vi "log.write.request.vi"(6 "Channel":string, 8 "error in":errorcluster, 9 "Arguments":map{string, string}(c390), 10 "Message":string, 11 "Time Stamp (now: system time)":timestamp format="%<%x %.3X>T") -> (0 "error out":errorcluster, 3 "request":string)   [LabVIEW 2020, in "Nominal Client.lvclass"]
uses:
  Nominal Client.lvclass
  8accc981-0023-4d42-bd6a-63233f6e5657.vi
  4260bc31-df4d-47d5-a4e2-998131efb0a5.vi
  bb59544d-9623-4990-916d-6c8c801fc026.vi
  9ae5cbee-81e9-4394-a3ea-0608fb529230.vi
  <vilib>/LabVIEW Open Source Project/Epoch Date & Time/epoch.UNIX/Epoch.UNIX.lvclass
  C:/Program Files (x86)/National Instruments/LabVIEW 2020/vi.lib/LabVIEW Open Source Project/Epoch Date & Time/epoch/Epoch.lvclass
  <vilib>/LabVIEW Open Source Project/Epoch Date & Time/Get Epoch Time.vi
  <vilib>/JDP Science/JSONtext/Variant to JSON Text.vi
  <vilib>/JDP Science/JSONtext/support/Format JSON Object.vi
  <vilib>/JDP Science/JSONtext/support/Format JSON Array Text.vi
  <vilib>/JDP Science/JSONtext/LVClass Serializer/JSONtext LVClass Serializer.lvclass
  nominal types/properties/properties.lvclass
  <vilib>/JDP Science/JSONtext/JSONtext.lvlib
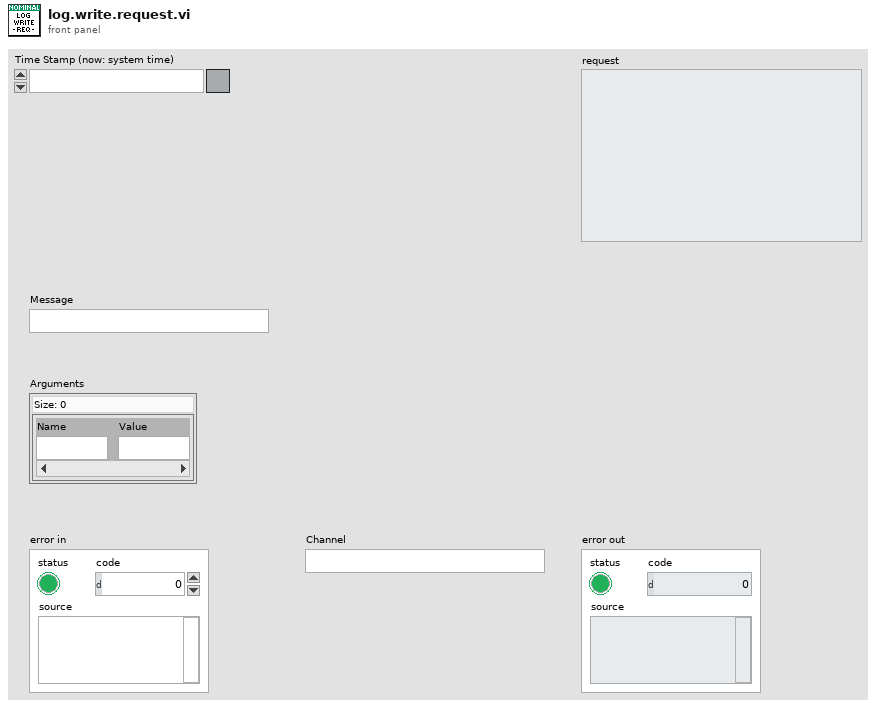
[diagram p1: front panel]
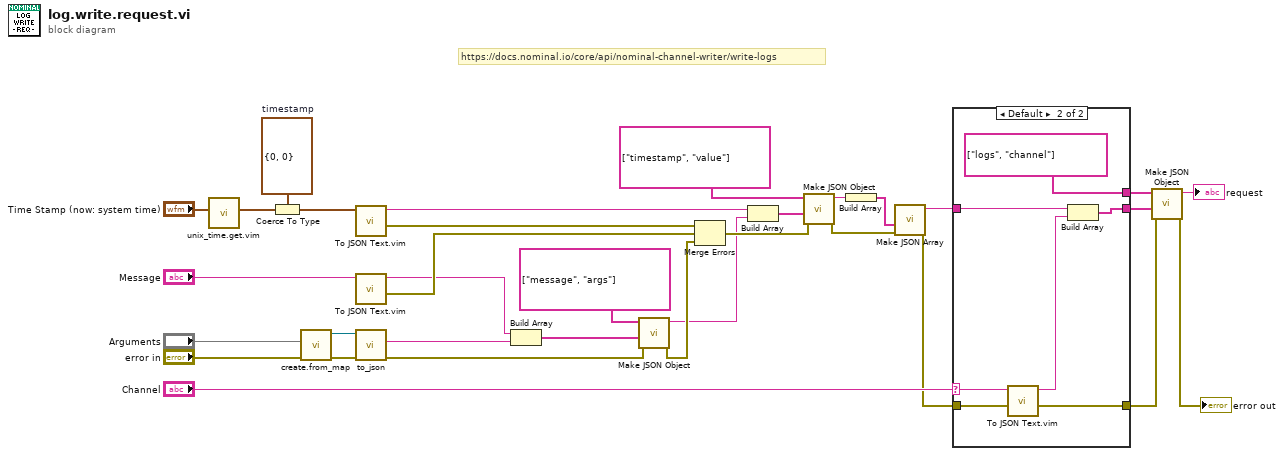
[diagram p0: block diagram]
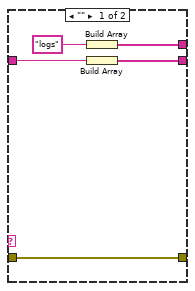
[diagram p2: hidden frame]
diagram:
  w32 = cluster{"seconds":i32, "nanos":i32} {"seconds"=0, "nanos"=0}  # timestamp
  # "https://docs.nominal.io/core/api/nominal-channel-writer/write-logs"
  n1 = call "unix_time.get.vim"("Time Stamp (empty: now) [single or array]"="Time Stamp (now: system time)") -> ("UNIX Timestamp"=w33:cluster{"Seconds":i64, "Nanoseconds":i64})  [unwired: 10 in]
  n2 = Coerce To Type(0:w33, 1:w32) -> (2:w28:cluster{"seconds":i32, "nanos":i32})
  n3 = call "create.from_map.vi"("error in"="error in", "properties"="Arguments") -> ("error out"=w29:errorcluster, "properties out"=w30:refnum<class "properties.lvclass">)  [unwired: 8 in]
  n4 = call "To JSON Text.vim"("Anything"=w28) -> ("error out"=w19:errorcluster, "<JSON>"=w23:string)  [unwired: 9 in]
  n5 = call "To JSON Text.vim"("Anything"="Message") -> ("error out"=w18:errorcluster, "<JSON>"=w14:string)  [unwired: 9 in]
  n6 = call-dynamic "to_json.vi"("error in"=w29, "properties in"=w30) -> ("error out"=w20:errorcluster, "json"=w26:string)  [unwired: 6 in, 2 out]
  n7 = Build Array(w14, w26) -> (w25:string[])
  n8 = call <vilib>:"Make JSON Object.vi"("error in (no error)"=w20, "JSON Items"=w25, "Item Names"=string[] ["message", "args"]) -> ("error out"=w17:errorcluster, "<JSON>"=w15:string)  [unwired: 7 in]
  n9 = Merge Errors(w19, w18, w17) -> (w16:errorcluster)
  n10 = Build Array(w23, w15) -> (w22:string[])
  n11 = call <vilib>:"Make JSON Object.vi"("error in (no error)"=w16, "JSON Items"=w22, "Item Names"=string[] ["timestamp", "value"]) -> ("error out"=w6:errorcluster, "<JSON>"=w9:string)  [unwired: 7 in]
  n12 = Build Array(w9) -> (w10:string[])
  n13 = call <vilib>:"Make JSON Array.vi"("error in (no error)"=w6, "JSON Elements"=w10) -> ("error out"=w7:errorcluster, "<JSON>"=w8:string)  [unwired: 8 in]
  n14 = case shown="Default" "Channel" {
    selector: "Channel" -> [_ w45]
    tunnel: w8 -> [w38 w44]
    tunnel: w7 -> [w34 w40]
    tunnel: [w35 string[] ["logs", "channel"] ("string")] -> w5
    tunnel: [w37 w41] -> w4
    tunnel: [w34 w39] -> w1
    frame "" {
      n15 = Build Array("logs" ("string")) -> (w35:string[])
      n16 = Build Array(w38) -> (w37:string[])
    }
    frame Default {
      n17 = call "To JSON Text.vim"("error in (no error)"=w40, "Anything"=w45) -> ("error out"=w39:errorcluster, "<JSON>"=w43:string)  [unwired: 8 in]
      n18 = Build Array(w44, w43) -> (w41:string[])
    }
  }
  n19 = call <vilib>:"Make JSON Object.vi"("error in (no error)"=w1, "JSON Items"=w4, "Item Names"=w5) -> ("error out"=→"error out":errorcluster, "<JSON>"=→"request":string)  [unwired: 7 in]
